vi "SetOverCurrProtLimit.vi"(3 "error in (no error)":errorcluster, 4 "Current":dbl, 5 "VISA resource name":refnum<visa-resource-name>) -> (0 "error out":errorcluster, 2 "VISA resource name out":refnum<visa-resource-name>)   [LabVIEW 2019, in "9103Series.lvlib"]
uses:
  <instrlib>/9103series/9103Series.lvlib
panel:
  out "ok?":string
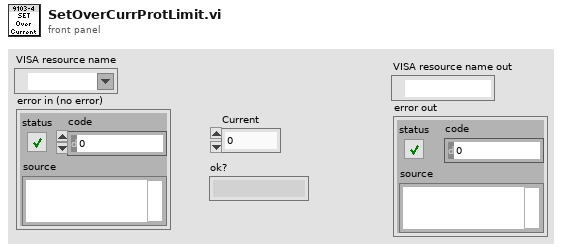
[diagram p1: front panel]
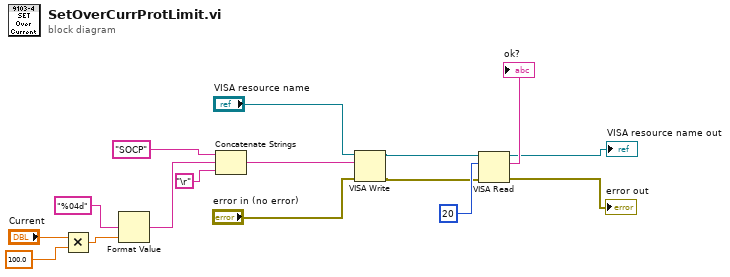
[diagram p0: block diagram]
diagram:
  n1 = Multiply(x="Current", y=100.0) -> (x*y=w9:dbl)
  n2 = Format Value(format string="%04d", value (0)=w9) -> (output string=w14:string)  [unwired: 1 in]
  n3 = Concatenate Strings("SOCP" ("string"), w14, "\r") -> (w11:string)
  n4 = VISA Write(VISA resource name="VISA resource name", write buffer=w11, error in (no error)="error in (no error)") -> (VISA resource name out=w3:refnum<visa-resource-name>, error out=w2:errorcluster)  [unwired: 1 out]
  n5 = VISA Read(VISA resource name=w3, byte count=u32 20, error in (no error)=w2) -> (VISA resource name out=→"VISA resource name out":refnum<visa-resource-name>, read buffer=→"ok?":string, error out=→"error out":errorcluster)  [unwired: 1 out]
